vi "EEG_2022_040_LabView_6.2.vi"() -> ()   [LabVIEW 2022 SP3]
panel:
  out "Temperature History":cluster{ext, "Temperature":dbl}(graph)
  in  "stop":bool
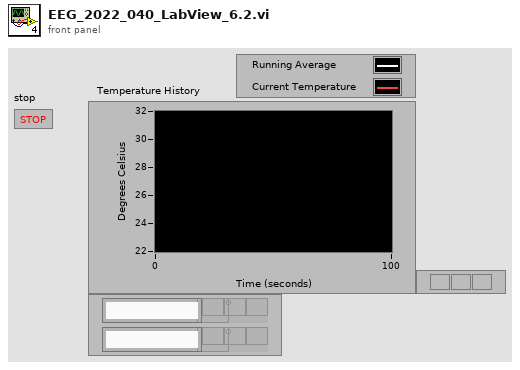
[diagram p1: front panel]
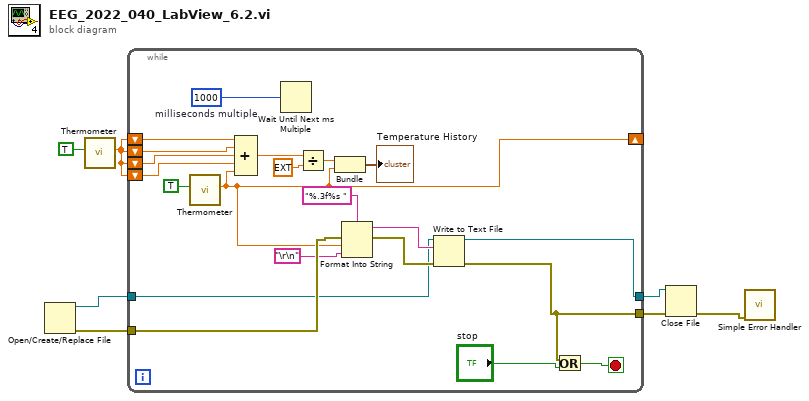
[diagram p0: block diagram]
diagram:
  n1 = Open/Create/Replace File() -> (refnum out=w5:refnum<file>, error out=w3:errorcluster)  [unwired: 6 in, 1 out]
  n2 = call "Thermometer.vi"("Temp Scale"=TRUE) -> ("Temperature"=w7:dbl)  [unwired: 9 in, 1 out]
  n3 = while {
    shift-right: [w9] -> _
    shift-left: w7 -> [w22]
    shift-left: w7 -> [w23]
    shift-left: w7 -> [w24]
    shift-left: w7 -> [w25]
    tunnel: [w14] -> w4
    tunnel: w5 -> [w15]
    tunnel: w3 -> [w18]
    tunnel: [w12] -> w2
    stop <- w11 stop-if-true
    w28 = 1000  # milliseconds multiple
    n4 = call "Thermometer.vi"("Temp Scale"=TRUE) -> ("Temperature"=w9:dbl)  [unwired: 9 in, 1 out]
    n5 = Compound Arithmetic op=ADD(w25, w24, w23, w22, w9) -> (w27:dbl)
    n6 = Wait Until Next ms Multiple(millisecond multiple=w28) -> ()  [unwired: 1 out]
    n7 = Divide(x=w27, y=ext 5.0) -> (x/y=w20:ext)
    n8 = Bundle(w20, "Temperature"=w9) -> (→"Temperature History":cluster{ext, "Temperature":dbl})  [unwired: 1 in]
    n9 = Format Into String(format string="%.3f%s ", error in=w18, w9, "\r\n") -> (resulting string=w17:string, error out=w16:errorcluster)  [unwired: 1 in]
    n10 = Write to Text File(file (use dialog)=w15, text=w17, error in=w16) -> (refnum out=w14:refnum<file>, error out=w12:errorcluster)  [unwired: 1 in, 1 out]
    n11 = Or(x=w12, y="stop") -> (x .or. y?=w11:bool)
  }
  n12 = Close File(refnum=w4, error in=w2) -> (error out=w1:errorcluster)  [unwired: 1 out]
  n13 = call <vilib>:"Simple Error Handler.vi"("error in (no error)"=w1) -> ()  [unwired: 4 in, 5 out]
